vi "Entry.vi"(8 "error in (no error)":errorcluster, 11 "New State":refnum<class "State.lvclass">) -> (0 "error out":errorcluster, 3 "State out":refnum<class "State.lvclass">)   [LabVIEW 2024, in "State.lvlib" / "State.lvclass"]
doc: "This is an abstract method. Override this method to define the behavior when you enter the state."
uses:
  State.lvclass
  State.lvclass/State.ctl
  <vilib>/NI/Actors/State Actor/State Actor/State Actor.lvclass
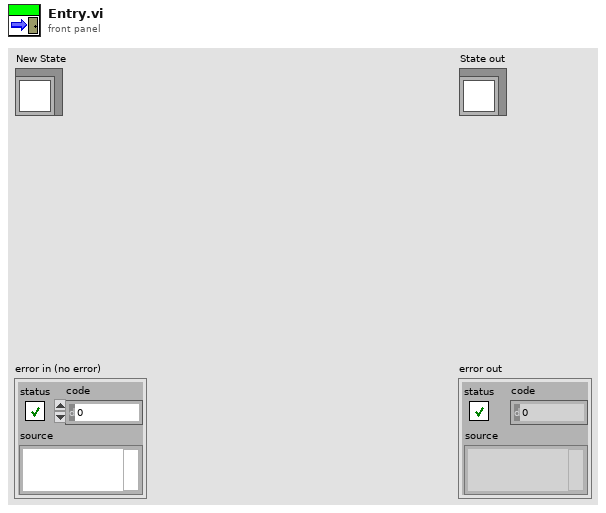
[diagram p1: front panel]
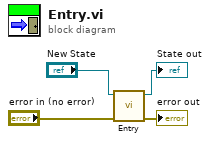
[diagram p0: block diagram]
diagram:
  n1 = call-parent "Entry.vi"("error in (no error)"="error in (no error)", "New State"="New State") -> ("error out"=→"error out":errorcluster, "State out"=→"State out":refnum<class "State.lvclass">)  [unwired: 8 in]
